vi "Initialize.vi"(8 "error in":errorcluster, 10 "parameters":variant, 11 "DMM Instrument in":refnum<class "DMM Instrument.lvclass">) -> (0 "error out":errorcluster, 2 "summary":T1(array[cluster]), 3 "data value reference":refnum<data-value>)   [LabVIEW 2025, in "DMM.lvlib" / "DMM Instrument.lvclass"]
doc: "Initializes the data of a node to its default state.\nThe object is not created inside of this VI, because it is created from a File depending on user selection.\nCopyright 2017 National Instruments Corporation\n\nLicensed under the Apache License, Version 2.0 (the \"License\"); you may not use this file except in compliance with the License. You may obtain a copy of the License at http://www.apache.org/licenses/LICENSE-2.0\nUnless required by applicable law or agreed to in writing, software distributed under the License is distributed on an \"AS IS\" BASIS, WITHOUT WARRANTIES OR CONDITIONS OF ANY KIND, either express or implied. See the License for the specific language governing permissions and limitations under the License."
uses:
  DMM Instrument.lvclass
  Users/Public/Documents/Sandia National Labs/TSS Plugin/CEF.lvlibp/Node/CEF_Node.lvclass
  DMM Instrument.lvclass/DMM Instrument.ctl
  DMM configuration/DMM configuration.lvclass
  C:/Users/Public/Documents/Sandia National Labs/TSS Plugin/Abstract Engine.lvlibp/Plugin/Abstract/Instrument configuration/Instrument configuration.lvclass
  Users/Public/Documents/Sandia National Labs/TSS Plugin/Abstract Engine.lvlibp/Plugin/Abstract/Instrument configuration/Read Instrument Setting.vi
  Users/Public/Documents/Sandia National Labs/TSS Plugin/Abstract Engine.lvlibp/Plugin/Abstract/Instrument configuration/Write Instrument Setting.vi
  Users/Public/Documents/Sandia National Labs/TSS Plugin/Abstract Engine.lvlibp/Plugin/Abstract/Abstract Instrument/Abstract Instrument.lvclass
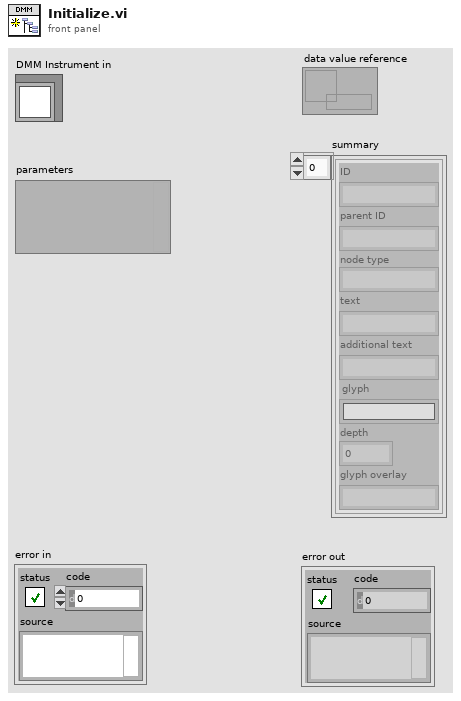
[diagram p1: front panel]
types:
  T1 = cluster{"ID":string, "parent ID":string, "node type":string, "text":string, "additional text":string, "glyph":string, "depth":i32, "glyph overlay":string}[]
  T2 = typedef "Abstract Engine.lvlibp/Instrument configuration.lvclass/Default Instrument.ctl" = cluster{"Type":string, "Address":string, "SW Alias":string, "Description":string, "Enabled":bool}
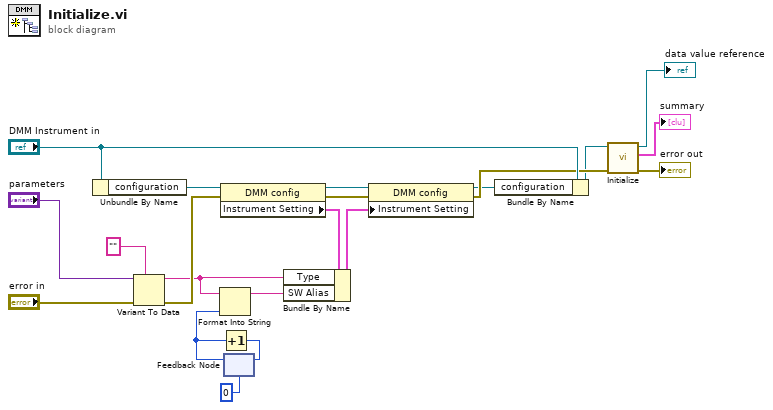
[diagram p0: block diagram]
diagram:
  n1 = Unbundle By Name("DMM Instrument in") -> ("configuration"=w16:refnum<class "DMM configuration.lvclass">)
  n2 = Variant To Data(error in="error in", type="", Variant="parameters") -> (data=w1:string, error out=w3:errorcluster)
  n3 = property class="DMM config"(reference=w16, error in=w3) -> (reference out=w15:refnum<class "DMM configuration.lvclass">, error out=w12:errorcluster, "Instrument Setting"=w14:T2)
  n4 = feedback #1(0) -> (w6:i32)
  n5 = Format Into String(initial string=w1, w6) -> (resulting string=w7:string)  [unwired: 2 in, 1 out]
  n6 = Increment(x=w6) -> (x+1=w4:i32)
  n7 = feedback-in #1(w4) -> ()
  n8 = Bundle By Name(cluster=w14, "Type"=w1, "SW Alias"=w7) -> (w13:T2)
  n9 = property class="DMM config"(reference=w15, error in=w12, "Instrument Setting"=w13) -> (reference out=w10:refnum<class "DMM configuration.lvclass">, error out=w11:errorcluster)
  n10 = Bundle By Name(cluster="DMM Instrument in", "configuration"=w10) -> (w9:refnum<class "DMM Instrument.lvclass">)
  n11 = call-parent "Initialize.vi"("error in"=w11, "CEF_Serialize node in"=w9) -> ("error out"=→"error out":errorcluster, "summary"=→"summary":T1, "data value reference"=→"data value reference":refnum<data-value>)  [unwired: 7 in]
